vi "ex_4_10_zle.vi"() -> ()   [LabVIEW 2020]
panel:
  out "Match Array":string[](array[string])
  in  "Match":string
  in  "String":string
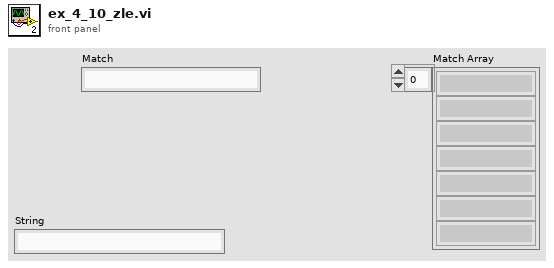
[diagram p1: front panel]
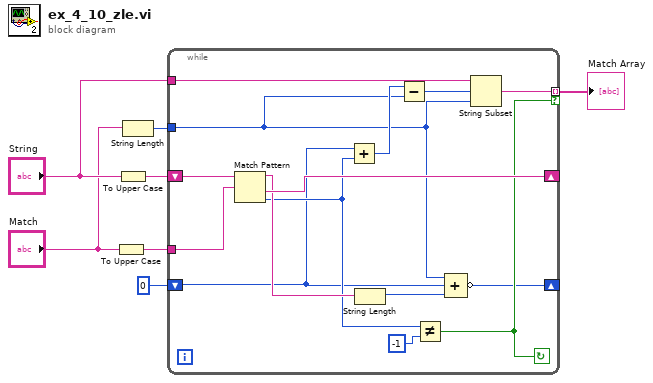
[diagram p0: block diagram]
diagram:
  n1 = To Upper Case(1:"Match") -> (0:w5:string)
  n2 = To Upper Case(1:"String") -> (0:w6:string)
  n3 = String Length(string="Match") -> (length=w3:i32)
  n4 = while {
    shift-right: [w20] -> _
    shift-left: w6 -> [w22]
    tunnel: w5 -> [w19]
    tunnel: [w16] -> w7 mode=indexing if=w18
    tunnel: "String" -> [w17]
    tunnel: w3 -> [w8]
    shift-right: [w11] -> _
    shift-left: 0 -> [w10]
    stop <- w18 continue-if-true
    n5 = Match Pattern(string=w22, regular expression=w19) -> (before substring=w14:string, after substring=w20:string, offset past match=w12:i32)  [unwired: 1 in, 1 out]
    n6 = Add(x=w10, y=w12) -> (x+y=w13:i32)
    n7 = String Length(string=w14) -> (length=w9:i32)
    n8 = Subtract(x=w13, y=w8) -> (x-y=w15:i32)
    n9 = Not Equal?(x=w12, y=-1) -> (x != y?=w18:bool)
    n10 = Compound Arithmetic op=ADD(w8, w10, w9) -> (invert w11:i32)
    n11 = String Subset(string=w17, offset (0)=w15, length (rest)=w8) -> (substring=w16:string)
  }
  "Match Array" <- w7
